vi "wait4noti.vi"(8 "error in (no error)":errorcluster, 11 "notifier":refnum<notifier>) -> (0 "error out":errorcluster, 3 "notifier out":refnum<notifier>)   [LabVIEW 2020]
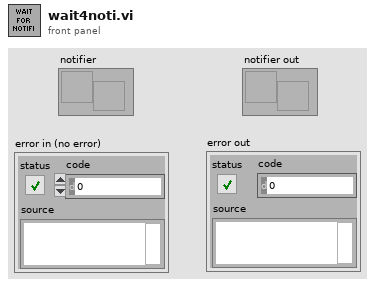
[diagram p1: front panel]
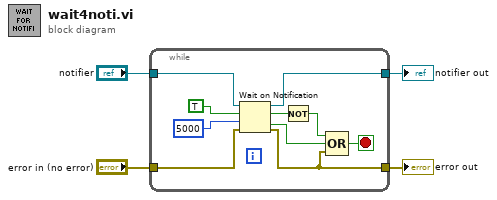
[diagram p0: block diagram]
diagram:
  n1 = while {
    tunnel: [w14] -> w2
    tunnel: "notifier" -> [w11]
    tunnel: [w6] -> w3
    tunnel: "error in (no error)" -> [w10]
    stop <- w5 stop-if-true
    n2 = Wait on Notification(notifier=w11, ignore previous (F)=TRUE, timeout in ms (-1)=5000, error in (no error)=w10) -> (notifier out=w14:refnum<notifier>, notification=w9:bool, timed out?=w7:bool, error out=w6:errorcluster)
    n3 = Not(x=w9) -> (.not. x?=w8:bool)
    n4 = Compound Arithmetic op=OR(w8, w7, w6) -> (w5:bool)
  }
  "error out" <- w3
  "notifier out" <- w2
